vi "call_MELEXIR.vi"(0 "Image Proc Directory":path=path "", 11 "error in (no error)":errorcluster, 13 "Controls":T1) -> (4 "PES Data Out":T2, 15 "error out":errorcluster)   [LabVIEW 2023]
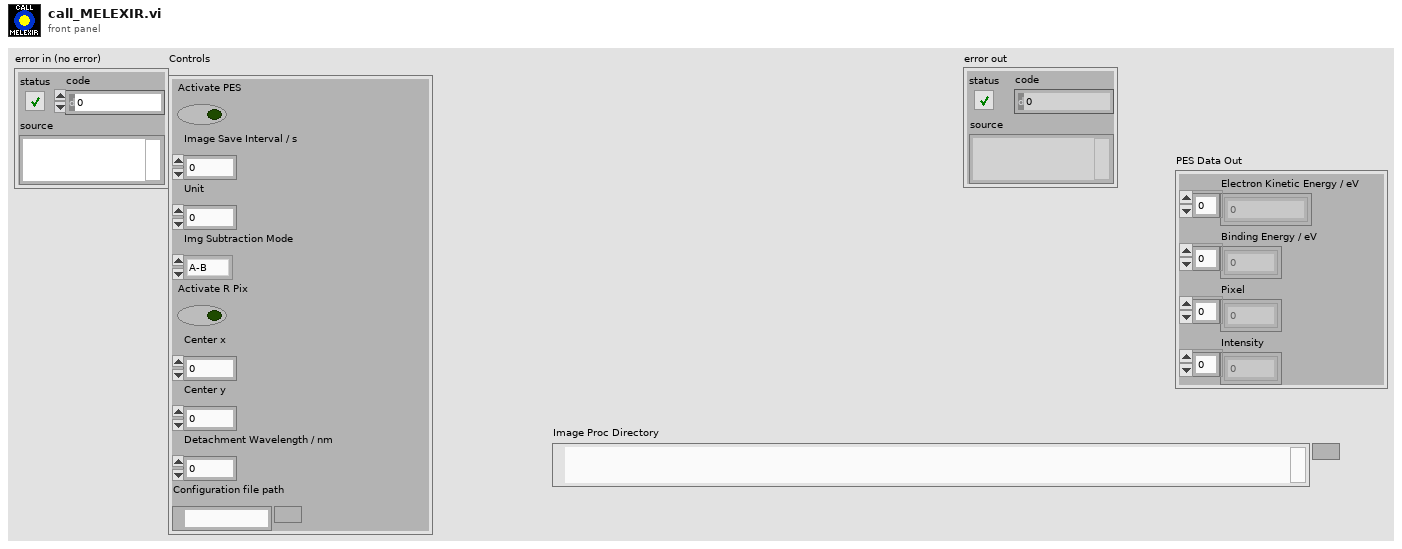
[diagram p1: front panel]
types:
  T1 = cluster{"Activate PES":bool, "Image Save Interval / s":dbl, "Unit":u16, "Img Subtraction Mode":enum16{"A-B", "B-A", "A+B"}, "Activate R Pix":bool, "Center x":i32, "Center y":i32, "Detachment Wavelength / nm":dbl, "Configuration file path":path}
  T2 = cluster{"Electron Kinetic Energy / eV":dbl[], "Binding Energy / eV":dbl[], "Pixel":dbl[], "Intensity":dbl[]}
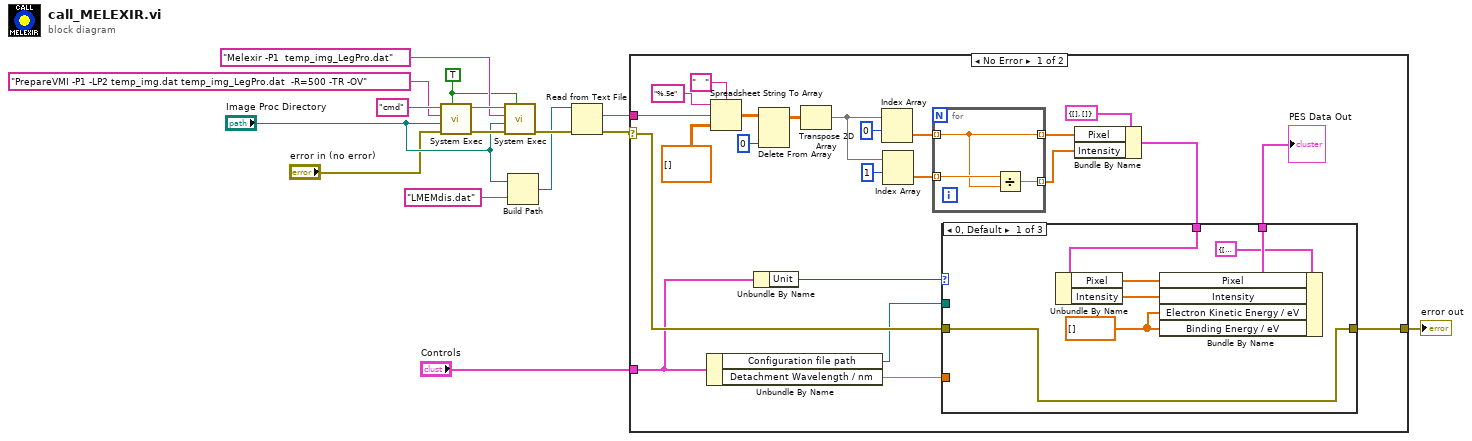
[diagram p0: block diagram]
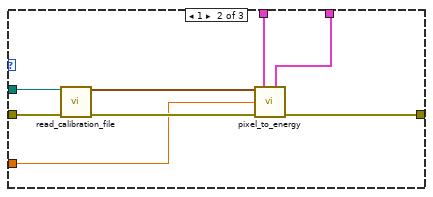
[diagram p2: hidden frame]
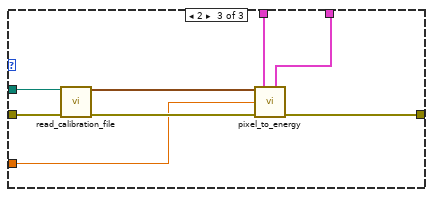
[diagram p3: hidden frame]
diagram:
  w4 = TRUE ("wait until completion? (T)")
  w13 = "cmd" ("command line")
  n1 = call <vilib>:"System Exec.vi"("wait until completion? (T)"=w4, "error in (no error)"="error in (no error)", "working directory"="Image Proc Directory", "standard input"="PrepareVMI -P1 -LP2 temp_img.dat temp_img_LegPro.dat  -R=500 -TR -OV", "command line"=w13) -> ("error out"=w14:errorcluster)  [unwired: 3 in, 3 out]
  n2 = call <vilib>:"System Exec.vi"("wait until completion? (T)"=w4, "error in (no error)"=w14, "working directory"="Image Proc Directory", "standard input"="Melexir -P1  temp_img_LegPro.dat", "command line"=w13) -> ("error out"=w8:errorcluster)  [unwired: 3 in, 3 out]
  n3 = Build Path(base path="Image Proc Directory", name or relative path="LMEMdis.dat" ("function name")) -> (appended path=w7:path)
  n4 = Read from Text File(file (use dialog)=w7, error in=w8) -> (text=w6:string, error out=w5:errorcluster)  [unwired: 2 in, 2 out]
  n5 = case shown="No Error" w5 {
    selector: w5 -> [w26 w64]
    tunnel: w6 -> [w37 _]
    tunnel: [w25 w64] -> w2
    tunnel: "Controls" -> [w16 _]
    frame No Error {
      n6 = Unbundle By Name(w16) -> ("Configuration file path"=w18:path, "Detachment Wavelength / nm"=w17:dbl)
      n7 = Spreadsheet String To Array(delimiter (Tab)="   ", format string="%.5e", spreadsheet string=w37, array type (2D Dbl)=dbl[][] []) -> (array=w34:dbl[][])
      n8 = Unbundle By Name(w16) -> ("Unit"=w15:u16)
      n9 = Delete From Array(array=w34, index (col)=0 ("disabled index (col)")) -> (array with subset deleted=w32:dbl[][])  [unwired: 2 in, 1 out]
      n10 = Transpose 2D Array(2D array=w32) -> (transposed array=w30:dbl[][])
      n11 = Index Array(array=w30, index (row)=0) -> (element=w28:dbl[])  [unwired: 1 in]
      n12 = Index Array(array=w30, index (row)=1) -> (element=w27:dbl[])  [unwired: 1 in]
      n13 = for {
        tunnel: w28 -> [w62] mode=indexing
        tunnel: w27 -> [w63] mode=indexing
        tunnel: [w62] -> w23 mode=indexing
        tunnel: [w61] -> w22 mode=indexing
        n14 = Divide(x=w63, y=w62) -> (x/y=w61:dbl)
      }
      n15 = Bundle By Name(cluster=cluster{"Pixel":dbl[], "Intensity":dbl[]} {"Pixel"=[], "Intensity"=[]}, "Pixel"=w23, "Intensity"=w22) -> (w21:cluster{"Pixel":dbl[], "Intensity":dbl[]})
      n16 = case shown="0, Default" w15 {
        tunnel: w26 -> [w42 w52 w60]
        tunnel: w18 -> [_ w51 w59]
        tunnel: [w42 w46 w54] -> w25
        tunnel: w21 -> [w41 w48 w56]
        tunnel: [w44 w47 w55] -> w20
        tunnel: w17 -> [_ w45 w53]
        frame 0, Default {
          w38 = dbl[] [] ("Intensity")
          n17 = Unbundle By Name(w41) -> ("Pixel"=w40:dbl[], "Intensity"=w39:dbl[])
          n18 = Bundle By Name(cluster=T2 {"Electron Kinetic Energy / eV"=[], "Binding Energy / eV"=[], "Pixel"=[], "Intensity"=[]} ("PES Data Out"), "Pixel"=w40, "Intensity"=w39, "Electron Kinetic Energy / eV"=w38, "Binding Energy / eV"=w38) -> (w44:T2)
        }
        frame 1 {
          n19 = call "read_calibration_file.vi"("configuration file path"=w51, "error in (no error)"=w52) -> ("Calibration Data"=w50:cluster{"quad_term":dbl, "linear_term":dbl}, "error out"=w49:errorcluster)  [unwired: 12 in]
          n20 = call "pixel_to_energy.vi"("Calibration Data"=w50, "PES Data In"=w48, "Detachment Wavelength / nm"=w45, "error in"=w49) -> ("PES Data Out"=w47:T2, "error out"=w46:errorcluster)  [unwired: 10 in]
        }
        frame 2 {
          n21 = call "read_calibration_file.vi"("configuration file path"=w59, "error in (no error)"=w60) -> ("Calibration Data"=w58:cluster{"quad_term":dbl, "linear_term":dbl}, "error out"=w57:errorcluster)  [unwired: 12 in]
          n22 = call "pixel_to_energy.vi"("Calibration Data"=w58, "PES Data In"=w56, "Detachment Wavelength / nm"=w53, "error in"=w57) -> ("PES Data Out"=w55:T2, "error out"=w54:errorcluster)  [unwired: 10 in]
        }
      }
      "PES Data Out" <- w20
    }
    frame Error {
    }
  }
  "error out" <- w2
